vi "Pumpstyrare.vi"() -> ()   [LabVIEW 2024]
panel:
  in  "stop":bool
  in  "MAX volym":dbl
  in  "MIN volym":dbl
  out "Waveform Chart":dbl(graph)
  in  "Propkonst (l/V)":dbl
  out "TOM":bool
  out "FULL":bool
  out "Tank":dbl(slide) scale=0.1..0.4
  in  "Samplingsintervall (ms)":i32
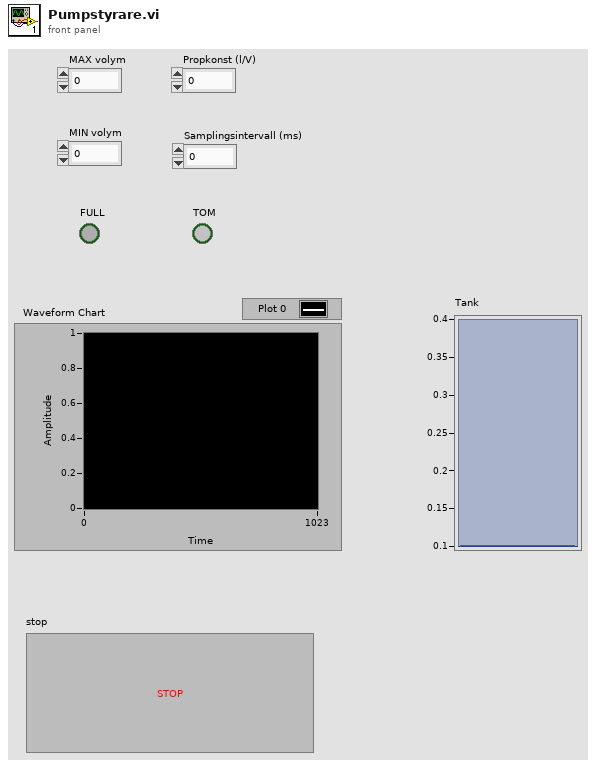
[diagram p1: front panel]
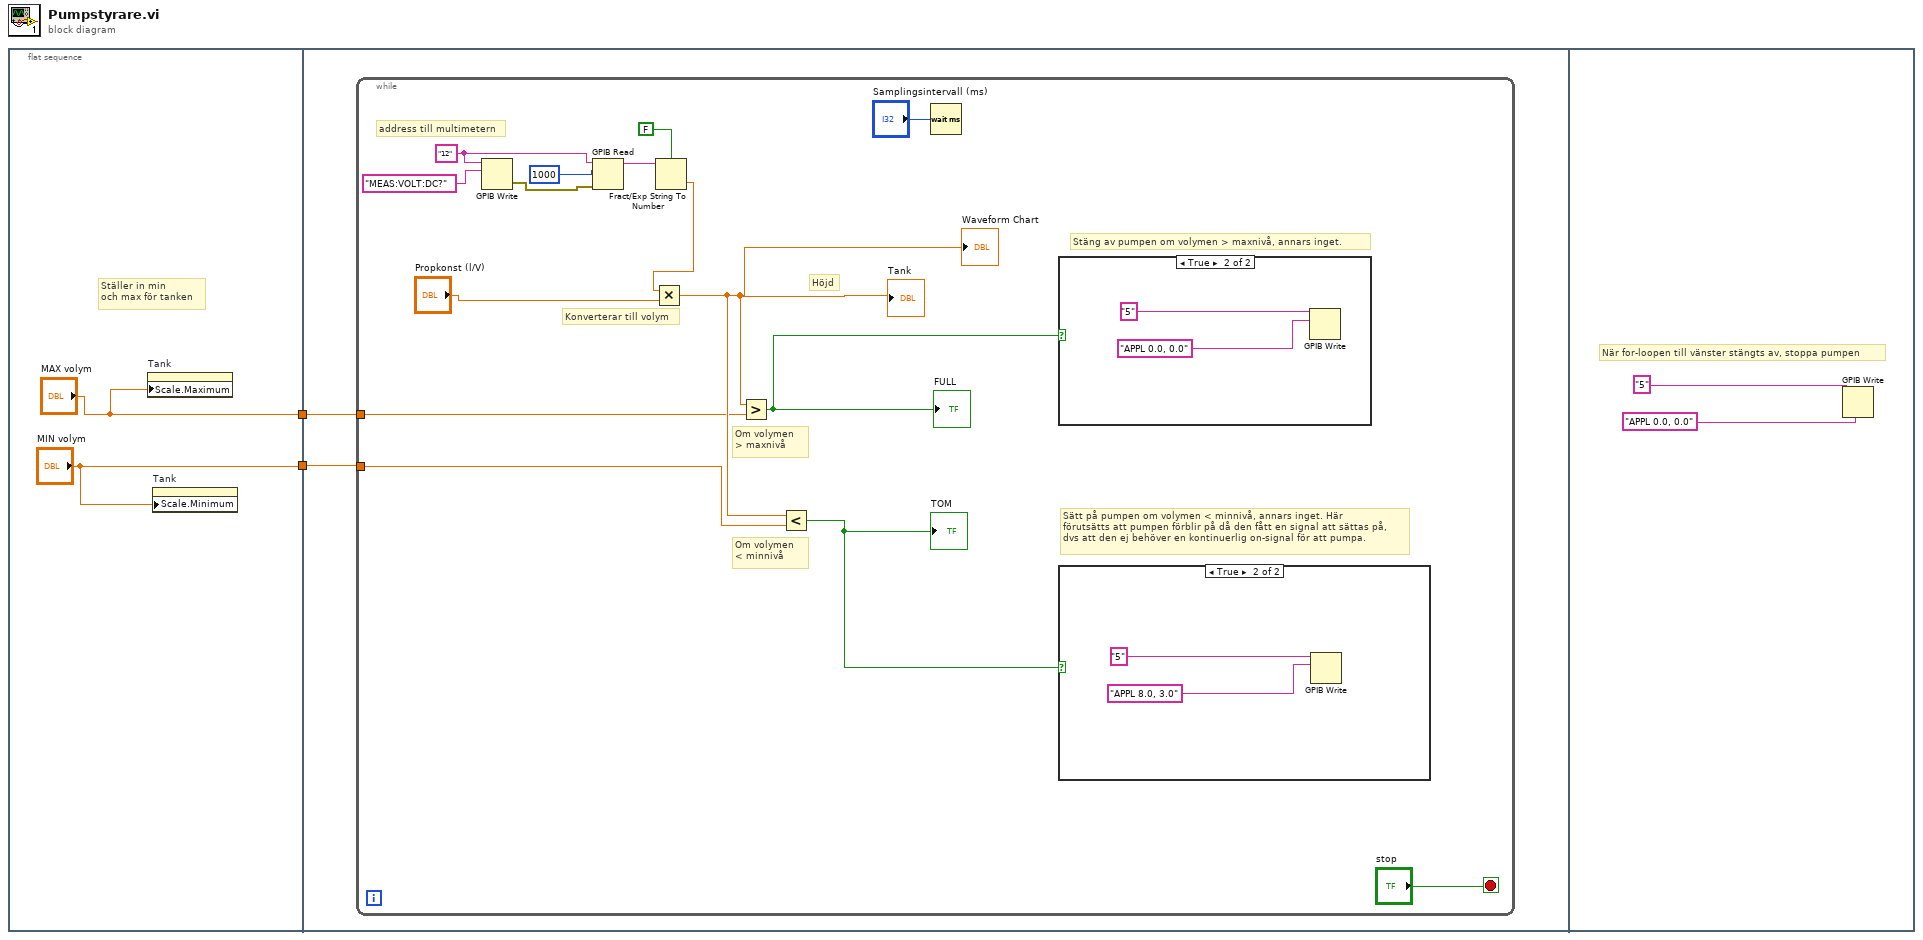
[diagram p0: block diagram]
diagram:
  n1 = flat-sequence {
    tunnel: ["MIN volym"] -> w2
    tunnel: ["MAX volym"] -> w1
    tunnel: w2 -> [w6]
    tunnel: w1 -> [w5]
    frame #0 {
      # "Ställer in min\noch max för tanken"
      n2 = property on="Tank" class="Slide (strict)"("Scale.Maximum"="MAX volym") -> ()  [unwired: 2 in, 2 out]
      n3 = property on="Tank" class="Slide (strict)"("Scale.Minimum"="MIN volym") -> ()  [unwired: 2 in, 2 out]
    }
    frame #1 {
      n4 = while {
        tunnel: w6 -> [w9]
        tunnel: w5 -> [w8]
        stop <- "stop" stop-if-true
        w20 = "12" ("address string")
        # "Om volymen \n< minnivå"
        # "Sätt på pumpen om volymen < minnivå, annars inget. Här\nförutsätts att pumpen förblir på då den fått en signal att sättas på,\ndvs att den ej behöver en kontinuerlig on-signal för att pumpa."
        # "Stäng av pumpen om volymen > maxnivå, annars inget."
        # "Om volymen \n> maxnivå"
        # "Höjd"
        # "Konverterar till volym"
        # "address till multimetern"
        n5 = GPIB Write(0:w20, 1:"MEAS:VOLT:DC?" ("data")) -> (6:w18:errorcluster)  [unwired: 3 in, 1 out]
        n6 = GPIB Read(0:w20, 1:1000 ("byte count"), 3:w18) -> (5:w16:string)  [unwired: 2 in, 2 out]
        n7 = Fract/Exp String To Number(use system decimal point (T)=FALSE, string=w16) -> (number=w15:dbl)  [unwired: 2 in, 1 out]
        n8 = Multiply(x=w15, y="Propkonst (l/V)") -> (x*y=w11:dbl)
        "Tank" <- w11
        "Waveform Chart" <- w11
        n9 = Greater?(x=w11, y=w8) -> (0:w13:bool)
        "FULL" <- w13
        n10 = Less?(x=w11, y=w9) -> (x < y?=w12:bool)
        "TOM" <- w12
        n11 = Wait (ms)(milliseconds to wait="Samplingsintervall (ms)") -> ()  [unwired: 1 out]
        n12 = case shown="True" w13 {
          frame False {
          }
          frame True {
            n13 = GPIB Write(0:"5" ("address string"), 1:"APPL 0.0, 0.0" ("data")) -> ()  [unwired: 3 in, 2 out]
          }
        }
        n14 = case shown="True" w12 {
          frame False {
          }
          frame True {
            n15 = GPIB Write(0:"5" ("address string"), 1:"APPL 8.0, 3.0" ("data")) -> ()  [unwired: 3 in, 2 out]
          }
        }
      }
    }
    frame #2 {
      # "När for-loopen till vänster stängts av, stoppa pumpen"
      n16 = GPIB Write(0:"5" ("address string"), 1:"APPL 0.0, 0.0" ("data")) -> ()  [unwired: 3 in, 2 out]
    }
  }
